vi "ME_acquire_3.vi"() -> ()   [LabVIEW 2015]
doc: "Use this template to build a producer/consumer design pattern. Use this template when you need to execute a process, such as data analysis, when a data source, such as a triggered acquisition, produces data at an uneven rate and you need to execute the process when the data becomes available."
uses:
  oxford_driver/Oxford Drivers/BUSGEN.LLB/OxfordAddress.ctl
  <vilib>/gmath/NI_Gmath.lvlib
  <vilib>/Utility/file.llb/Write Delimited Spreadsheet (DBL).vi
  <vilib>/express/express arith-compare/Formula/XNode/ExpressFormulaBlockNode.xnode
panel:
  out "I_dn_average":dbl[](array[numeric]) format="%_6g"
  out "I_dn_actual":dbl[](array[numeric]) format="%_6g"
  out "B array":dbl[](array[numeric])
  in  "dB (T)":dbl=0.0001
  in  "Counter":dbl
  out "I(B) 3":cluster{dbl[], dbl[]}(graph)
  out "I(B) 2":cluster{dbl[], dbl[]}(graph)
  out "I(B)":cluster{dbl[], dbl[]}(graph)
  in  "Max Field (T)":dbl
  in  "Min Field (T)":dbl
  in  "Ramp up/down":bool
  out "I_T":cluster{dbl[], dbl[]}(graph)
  in  "Field To Zero":bool
  in  "Set Field (T)":dbl=0.3
  in  "Go to Set":bool
  out "L magnet (H)":dbl
  out "R magnet (mOhm)":dbl
  out "Actual Current (R0)":dbl
  out "Actual Field (T)":dbl
  out "Set":bool
  in  "Target Sweep Rate (T/min)":dbl=2.0 format="%.6f"
  out "Temperature array":dbl[](array[numeric])
  in  "New Measurement File":bool
  out "Measurement File":path
  out "refnum out":refnum<file>
  in  "Sampling rate (Hz)":dbl=20.0
  in  "Measuring":bool
  out "Actual Temperature (K)":dbl
  in  "Temp Refresh (s)":dbl=1.0
  in  "Lake Shore":refnum<visa-resource-name>="GPIB0::11::INSTR"
  out "Time Lag":dbl=0.0500025749206543
  out "Magnetic Field":cluster{dbl[], dbl[]}(graph)
  out "IV converter":cluster{dbl[], dbl[]}(graph)
  in  "Measure (Start/Pause)":bool
  in  "Magnetic Field":refnum<visa-resource-name>="GPIB0::21::INSTR"
  in  "IV converter":refnum<visa-resource-name>="GPIB0::20::INSTR"
  in  "stop":bool
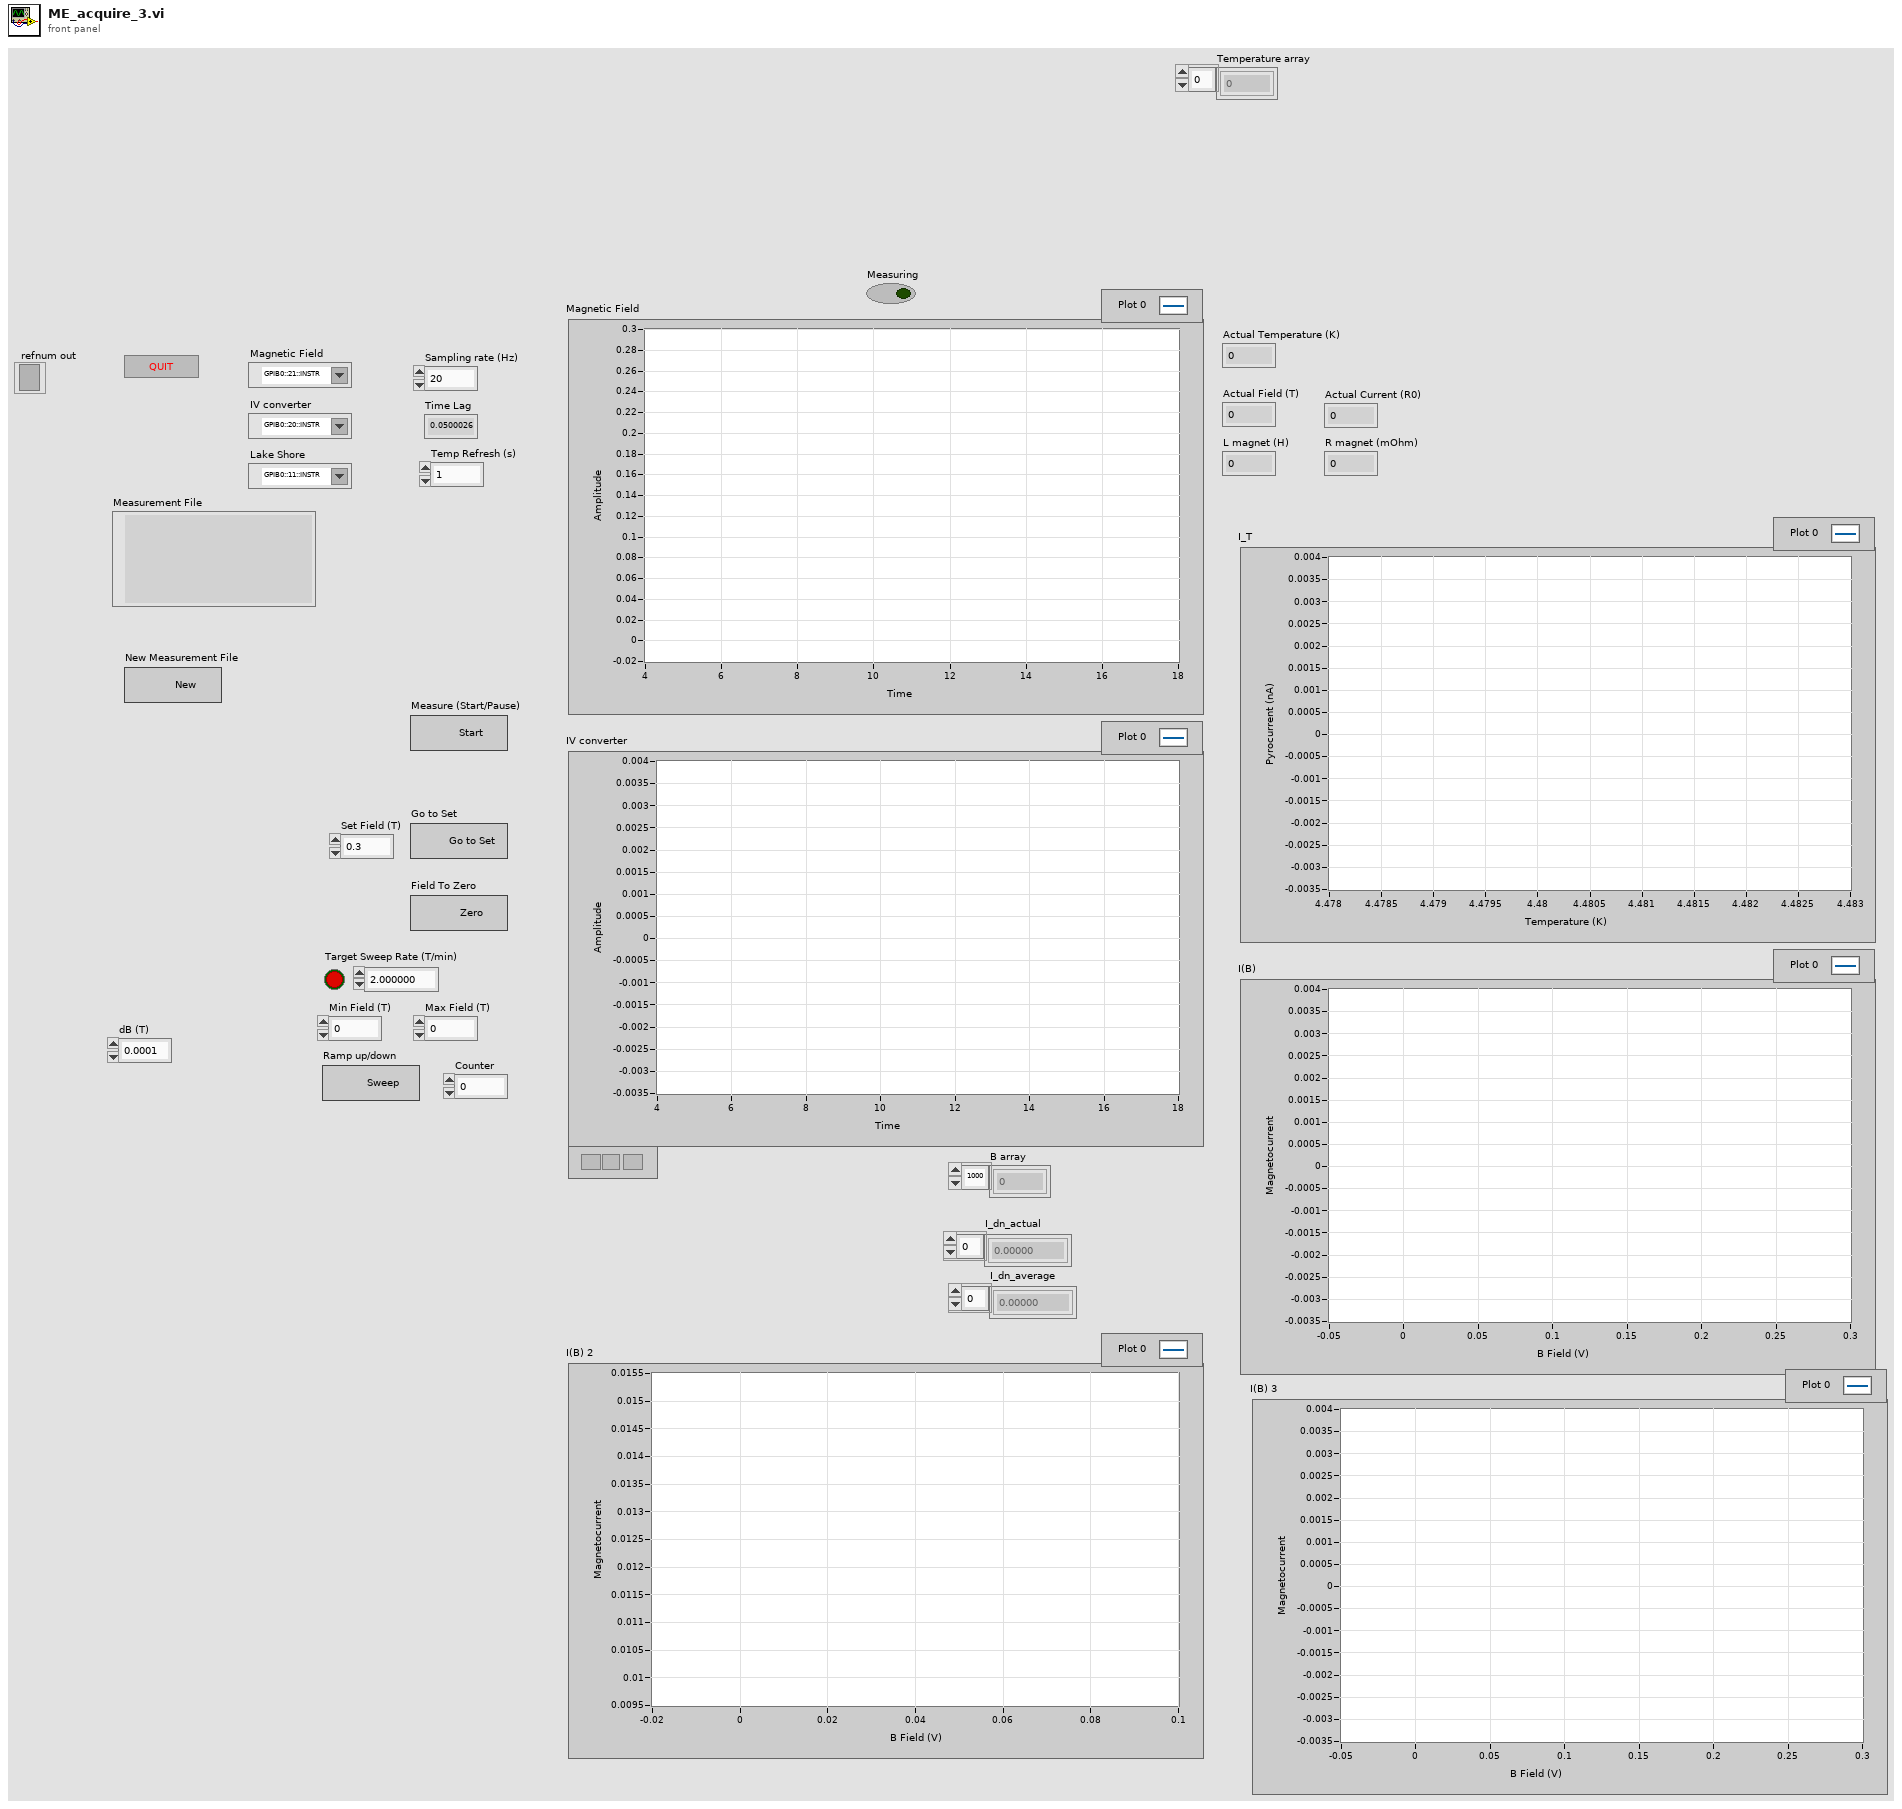
[diagram p1: front panel]
types:
  T1 = enum16{"open", "replace", "create", "open or create", "replace or create", "replace or create with confirmation"}
  T2 = typedef "OxfordAddress.ctl" = cluster{"Com Port":i32, "ISOBUS Address":i32, "GPIB Address":i16, "Communication":enum16{"RS232", "ISOBUS", "GPIB", "Gateway"}}
  T3 = cluster{"seconds since 1Jan1904":timestamp, "read buffer":string, "read buffer":string}
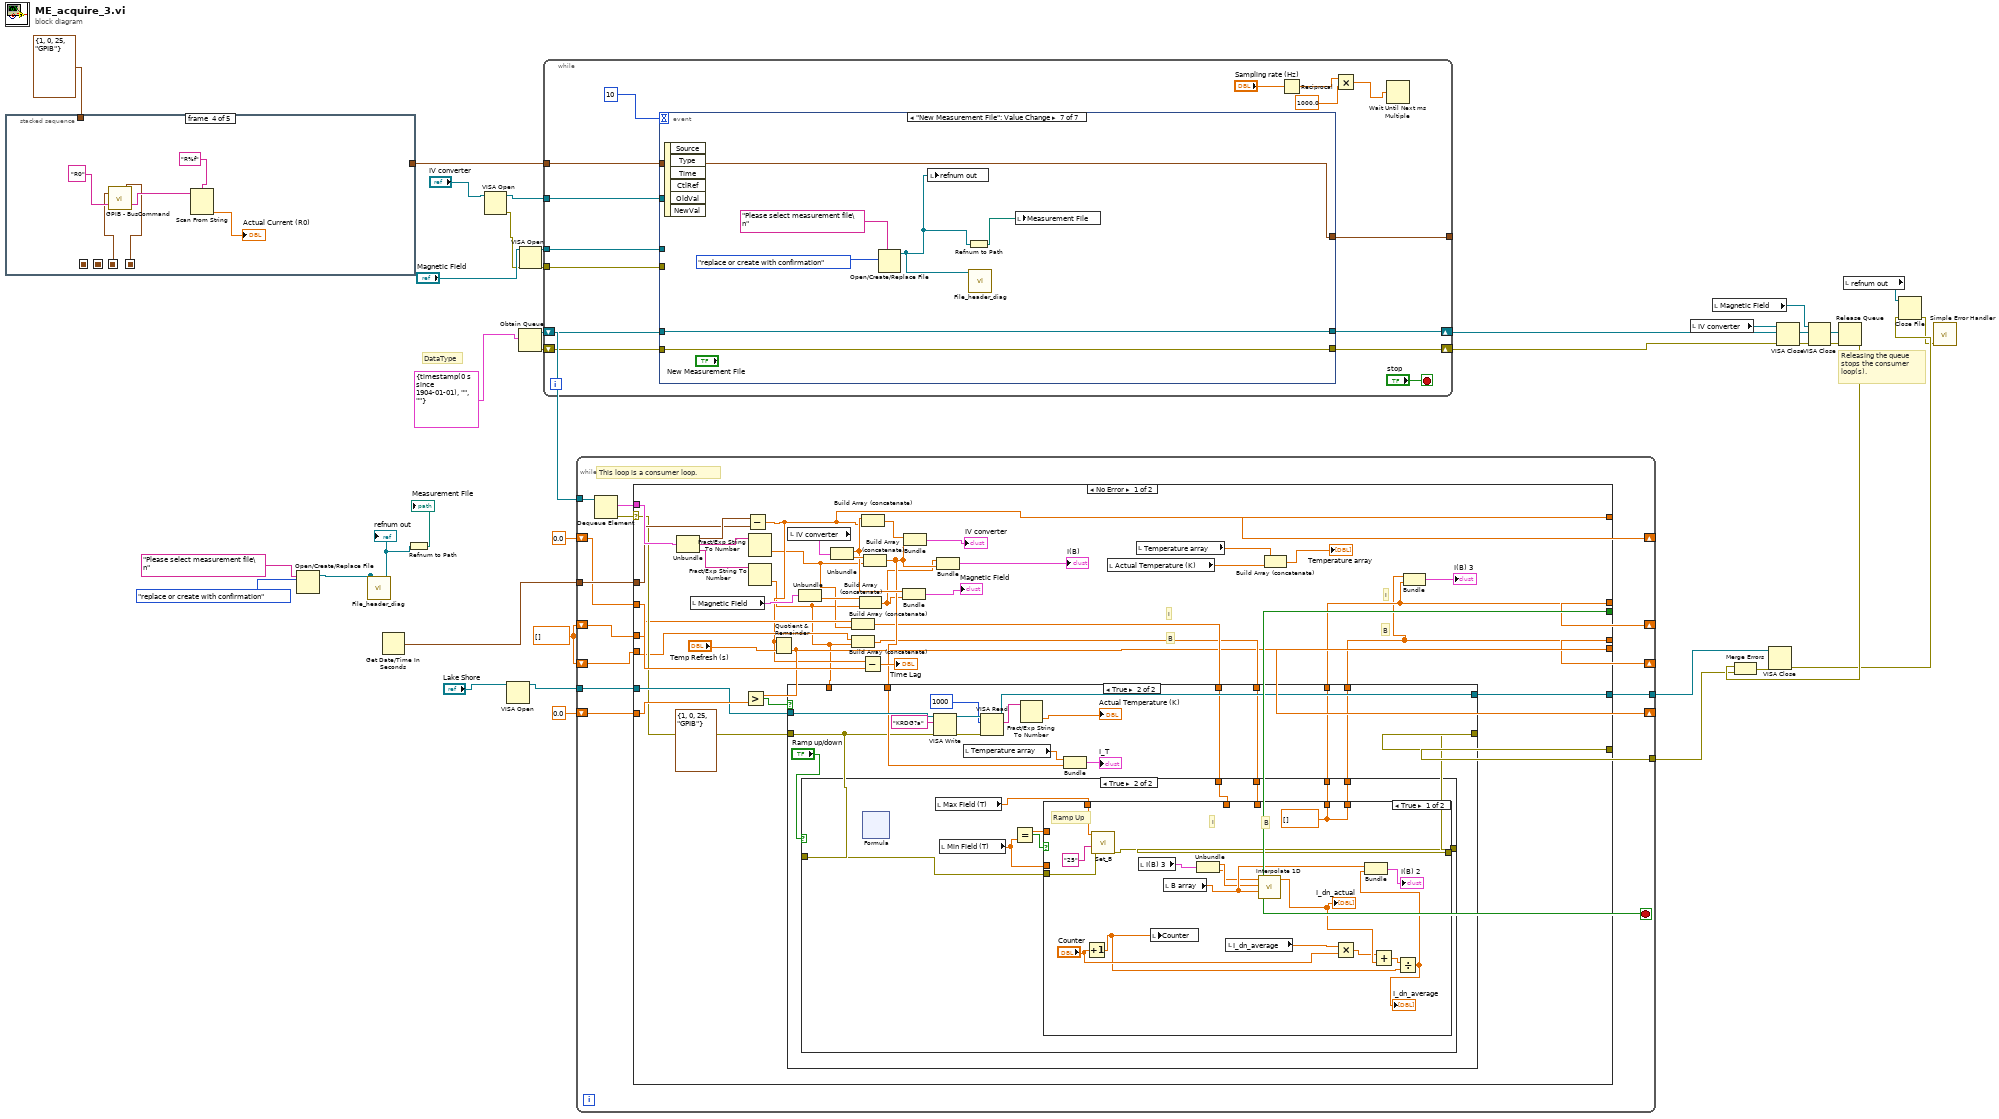
[diagram p0: block diagram]
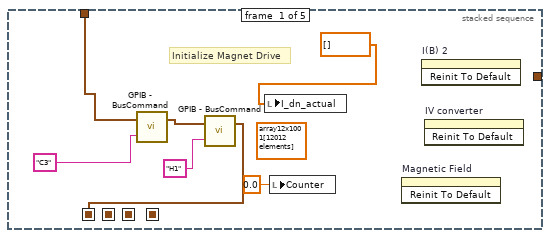
[diagram p2: hidden frame]
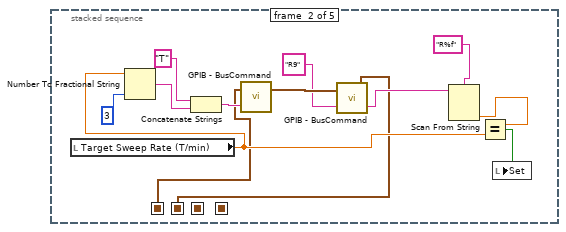
[diagram p3: hidden frame]
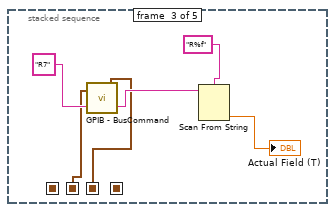
[diagram p4: hidden frame]
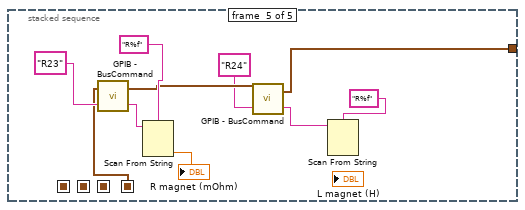
[diagram p5: hidden frame]
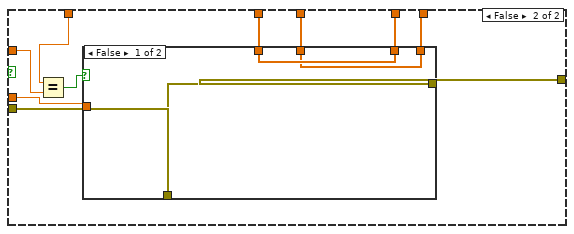
[diagram p8: hidden frame]
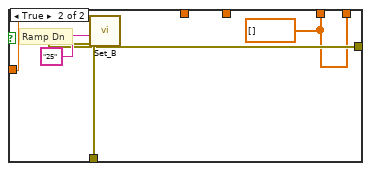
[diagram p9: hidden frame]
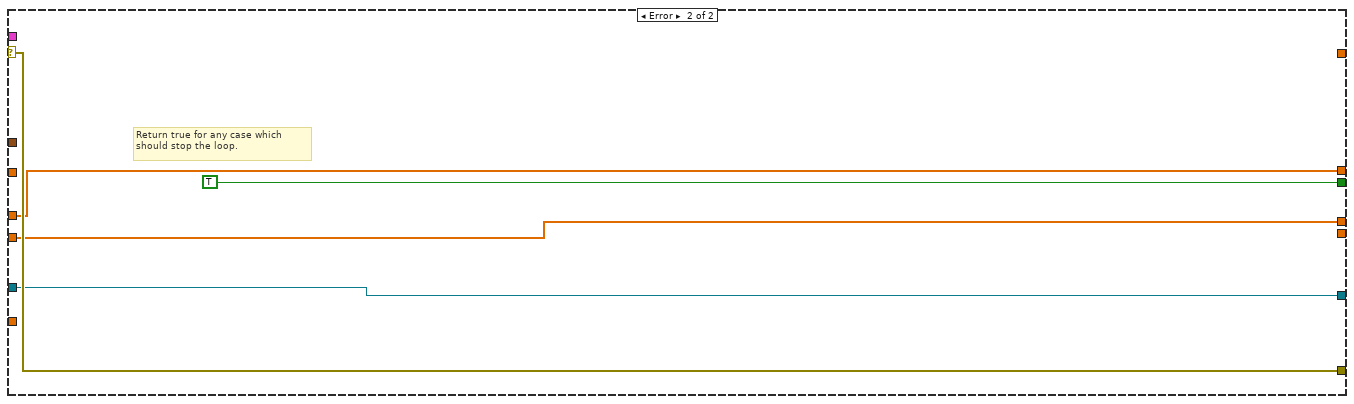
[diagram p10: hidden frame]
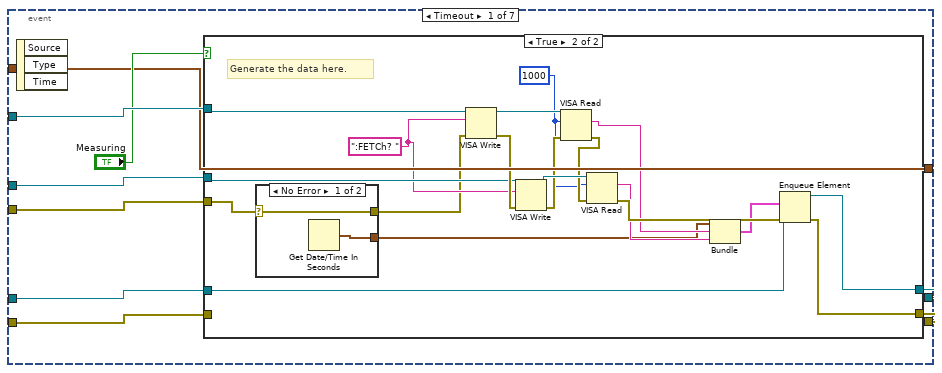
[diagram p11: hidden frame]
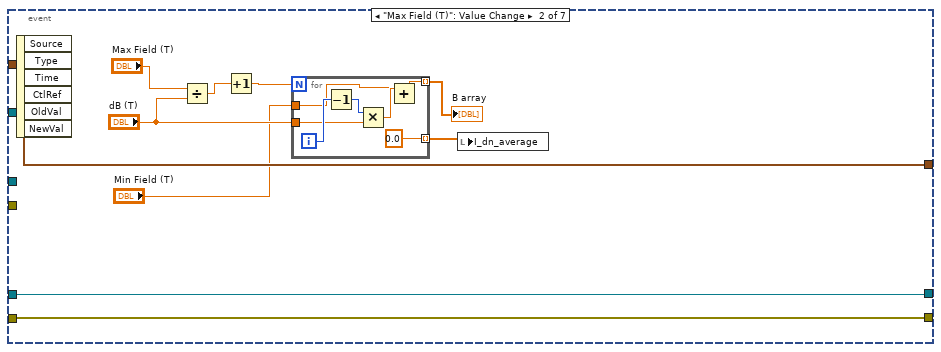
[diagram p14: hidden frame]
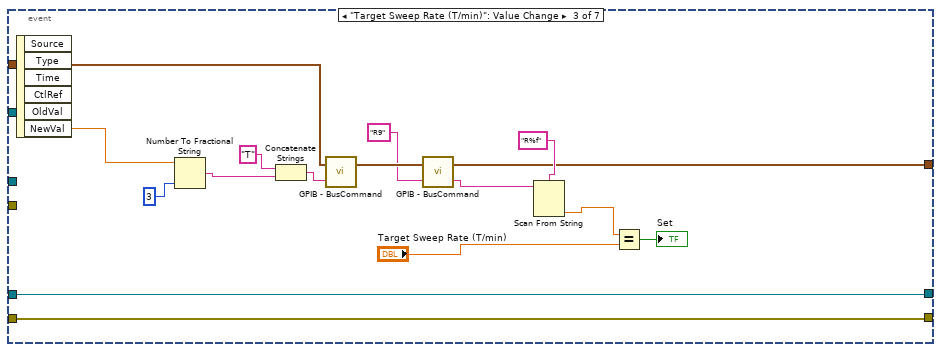
[diagram p15: hidden frame]
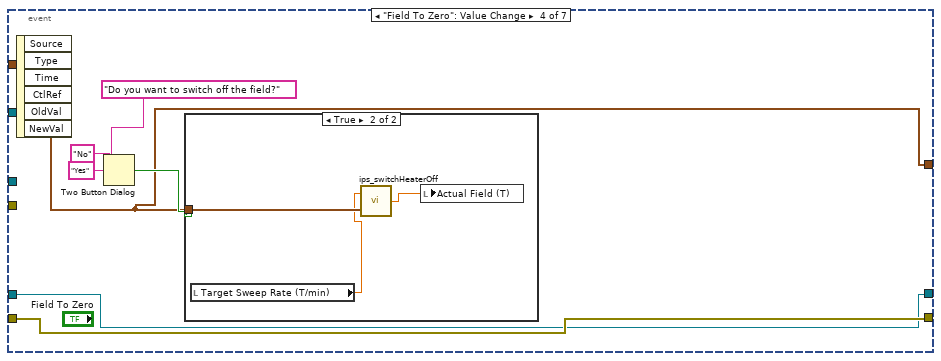
[diagram p16: hidden frame]
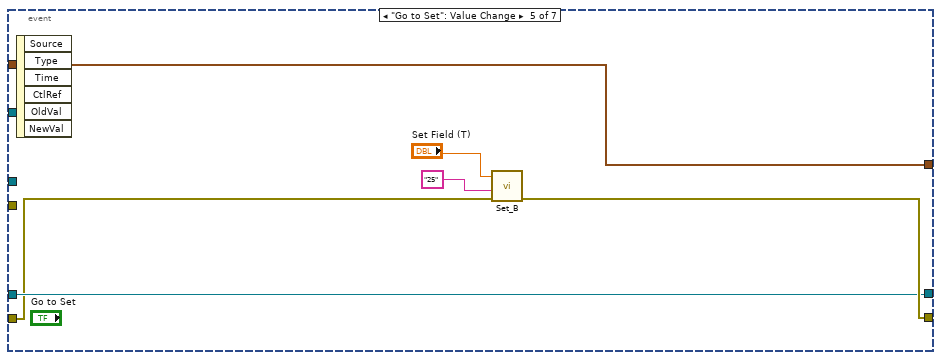
[diagram p18: hidden frame]
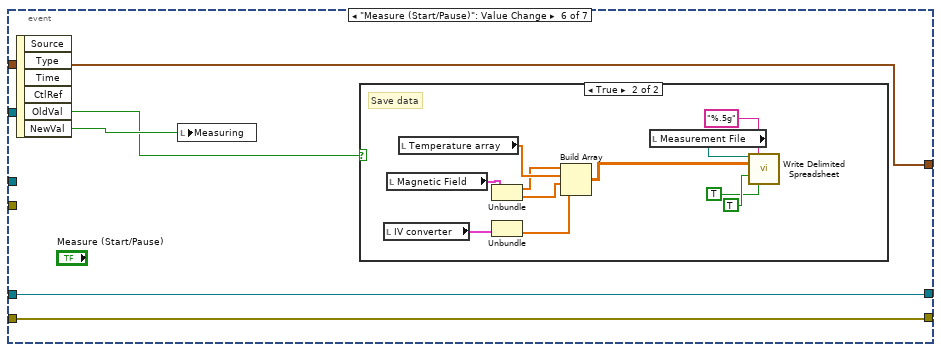
[diagram p19: hidden frame]
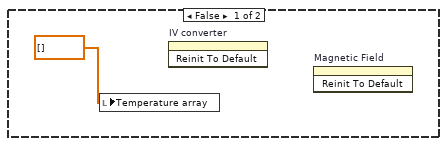
[diagram p20: hidden frame]
diagram:
  w5 = dbl[] []
  # "DataType"
  # "Releasing the queue stops the consumer loop(s)."
  n1 = stacked-sequence {
    seq-local: [w37 _ _ _ _] -> [_ w43 _ _ _]
    seq-local: [_ w42 _ _ _] -> [_ _ w56 _ _]
    seq-local: [_ _ w55 _ _] -> [_ _ _ w62 _]
    seq-local: [_ _ _ w61 _] -> [_ _ _ _ w72]
    tunnel: T2 {"Com Port"=1, "ISOBUS Address"=0, "GPIB Address"=25, "Communication"=enum."GPIB"} ("Address") -> [w40 _ _ _ _]
    tunnel: [_ _ _ _ w70] -> w6
    frame #0 {
      (unwired) dbl[][] array12x1001[12012 elements] ("I_dn_all")
      # "Initialize Magnet Drive"
      n2 = call "GPIB - BusCommand.vi"("Command"="C3", "Address"=w40) -> ("Address(thru)"=w38:T2)  [unwired: 1 out]
      n3 = call "GPIB - BusCommand.vi"("Command"="H1", "Address"=w38) -> ("Address(thru)"=w37:T2)  [unwired: 1 out]
      n4 = local write "I_dn_actual"(dbl[] [] ("Result")) -> ()
      n5 = local write "Counter"(0.0 ("Counter")) -> ()
      n6 = invoke on="Magnetic Field" class="XYGraph (strict)" method="Reinit To Default"() -> ()  [unwired: 3 in, 3 out]
      n7 = invoke on="I(B) 2" class="XYGraph (strict)" method="Reinit To Default"() -> ()  [unwired: 3 in, 3 out]
      n8 = invoke on="IV converter" class="XYGraph (strict)" method="Reinit To Default"() -> ()  [unwired: 3 in, 3 out]
    }
    frame #1 {
      n9 = local read "Target Sweep Rate (T/min)"() -> (w45:dbl)
      n10 = Number To Fractional String(number=w45, precision (6)=i16 3) -> (F-format string=w52:string)  [unwired: 2 in]
      n11 = Concatenate Strings("T" ("format string"), w52) -> (w51:string)
      n12 = call "GPIB - BusCommand.vi"("Command"=w51, "Address"=w43) -> ("Address(thru)"=w50:T2)  [unwired: 1 out]
      n13 = call "GPIB - BusCommand.vi"("Command"="R9" ("format string"), "Address"=w50) -> ("Reply"=w48:string, "Address(thru)"=w42:T2)
      n14 = Scan From String(format string="R%f" ("remaining string"), input string=w48) -> (output 1=w46:dbl)  [unwired: 3 in, 3 out]
      n15 = Equal?(x=w46, y=w45) -> (x = y?=w44:bool)
      n16 = local write "Set"(w44) -> ()
    }
    frame #2 {
      n17 = call "GPIB - BusCommand.vi"("Command"="R7" ("format string"), "Address"=w56) -> ("Reply"=w60:string, "Address(thru)"=w55:T2)
      n18 = Scan From String(format string="R%f" ("remaining string"), input string=w60) -> (output 1=→"Actual Field (T)":dbl)  [unwired: 3 in, 3 out]
    }
    frame #3 {
      n19 = call "GPIB - BusCommand.vi"("Command"="R0" ("format string"), "Address"=w62) -> ("Reply"=w66:string, "Address(thru)"=w61:T2)
      n20 = Scan From String(format string="R%f" ("remaining string"), input string=w66) -> (output 1=→"Actual Current (R0)":dbl)  [unwired: 3 in, 3 out]
    }
    frame #4 {
      n21 = call "GPIB - BusCommand.vi"("Command"="R23" ("format string"), "Address"=w72) -> ("Reply"=w76:string, "Address(thru)"=w71:T2)
      n22 = Scan From String(format string="R%f" ("remaining string"), input string=w76) -> (output 1=→"R magnet (mOhm)":dbl)  [unwired: 3 in, 3 out]
      n23 = call "GPIB - BusCommand.vi"("Command"="R24" ("format string"), "Address"=w71) -> ("Reply"=w68:string, "Address(thru)"=w70:T2)
      n24 = Scan From String(format string="R%f" ("remaining string"), input string=w68) -> ()  [unwired: 4 in, 3 out]
    }
  }
  n25 = Open/Create/Replace File(prompt="Please select measurement file\n", operation (0:open)=T1."replace or create with confirmation") -> (refnum out=w1:refnum<file>)  [unwired: 4 in, 2 out]
  "refnum out" <- w1
  n26 = call "File_header_diag.vi"("Byte Stream File in"=w1) -> ()  [unwired: 11 in]
  n27 = Get Date/Time In Seconds() -> (seconds since 1Jan1904=w19:timestamp)
  n28 = Refnum to Path(1:w1) -> (0:→"Measurement File":path)
  n29 = VISA Open(VISA resource name="IV converter") -> (VISA resource name=w28:refnum<visa-resource-name>, error out=w30:errorcluster)  [unwired: 4 in]
  n30 = VISA Open(VISA resource name="Lake Shore") -> (VISA resource name=w17:refnum<visa-resource-name>)  [unwired: 4 in, 1 out]
  n31 = Obtain Queue(element data type=T3 {"seconds since 1Jan1904"=timestamp(0 s since 1904-01-01), "read buffer"="", "read buffer"=""} ("output cluster")) -> (queue out=w34:refnum<queue>, error out=w33:errorcluster)  [unwired: 4 in, 1 out]
  n32 = VISA Open(error in (no error)=w30, VISA resource name="Magnetic Field") -> (VISA resource name=w27:refnum<visa-resource-name>, error out=w26:errorcluster)  [unwired: 3 in]
  n33 = while {
    shift-right: [w87] -> w24
    shift-left: w33 -> [w88]
    shift-right: [w89] -> w32
    shift-left: w34 -> [w90]
    tunnel: w28 -> [w86]
    tunnel: w27 -> [w85]
    tunnel: w26 -> [w84]
    tunnel: [w78] -> _
    tunnel: w6 -> [w77]
    stop <- "stop" stop-if-true
    n34 = event shown="[6] \"New Measurement File\": Value Change" {
      selector: _ -> [_ _ _ _ _ _ _]
      dyn-events: _ -> [_ _ _ _ _ _ _]
      timeout: 10 -> [_ _ _ _ _ _ _]
      tunnel: w90 -> [w100 w134 w143 w159 w170 w178 w192]
      tunnel: [w99 w134 w143 w159 w170 w178 w192] -> w89
      tunnel: w88 -> [w98 w133 w142 w160 w169 w177 w193]
      tunnel: [w97 w133 w142 w160 w171 w177 w193] -> w87
      tunnel: w86 -> [w96 _ _ _ _ _ _]
      tunnel: w85 -> [w95 _ _ _ _ _ _]
      tunnel: w84 -> [w94 _ _ _ _ _ _]
      tunnel: [w92 w132 w148 w158 w172 w174 w191] -> w78
      tunnel: w77 -> [w92 w132 w144 w158 w172 w174 w191]
      event Timeout {
        n35 = event-data() -> ()  [unwired: 1 in, 3 out]
        n36 = case shown="True" "Measuring" {
          tunnel: w100 -> [w102 w121]
          tunnel: [w102 w120] -> w99
          tunnel: w98 -> [w101 _]
          tunnel: [w101 w119] -> w97
          tunnel: w96 -> [_ w112]
          tunnel: w95 -> [_ w111]
          tunnel: w94 -> [_ w106]
          frame False {
          }
          frame True {
            w109 = ":FETCh? " ("data")
            w113 = u32 1000 ("byte count")
            # "Generate the data here."
            n37 = case shown="No Error" w106 {
              selector: w106 -> [w123 w124]
              tunnel: [w123 w124] -> w105
              tunnel: [w122 _] -> w104
              frame No Error {
                n38 = Get Date/Time In Seconds() -> (seconds since 1Jan1904=w122:timestamp)
              }
              frame Error {
              }
            }
            n39 = VISA Write(VISA resource name=w112, write buffer=w109, error in (no error)=w105) -> (VISA resource name out=w118:refnum<visa-resource-name>, error out=w116:errorcluster)  [unwired: 1 out]
            n40 = VISA Write(VISA resource name=w111, write buffer=w109, error in (no error)=w116) -> (VISA resource name out=w117:refnum<visa-resource-name>, error out=w115:errorcluster)  [unwired: 1 out]
            n41 = VISA Read(VISA resource name=w118, byte count=w113, error in (no error)=w115) -> (read buffer=w107:string, error out=w114:errorcluster)  [unwired: 2 out]
            n42 = VISA Read(VISA resource name=w117, byte count=w113, error in (no error)=w114) -> (read buffer=w108:string, error out=w110:errorcluster)  [unwired: 2 out]
            n43 = Bundle("seconds since 1Jan1904"=w104, "read buffer"=w107, "read buffer"=w108) -> (w103:T3)  [unwired: 1 in]
            n44 = Enqueue Element(queue=w121, element=w103, error in (no error)=w110) -> (queue out=w120:refnum<queue>, error out=w119:errorcluster)  [unwired: 1 in, 1 out]
          }
        }
      }
      event "Max Field (T)": Value Change {
        n45 = event-data() -> ()  [unwired: 1 in, 6 out]
        n46 = Divide(x="Max Field (T)", y="dB (T)") -> (x/y=w129:dbl)
        n47 = Increment(x=w129) -> (x+1=w128:dbl)
        n48 = for {
          N: w128 -> [_]
          tunnel: "dB (T)" -> [w139]
          tunnel: [w136] -> w127 mode=indexing
          tunnel: "Min Field (T)" -> [w137]
          tunnel: [0.0] -> w125 mode=indexing
          i -> [w141]
          n49 = Decrement(x=w141) -> (x-1=w140:i32)
          n50 = Multiply(x=w140, y=w139) -> (x*y=w138:dbl)
          n51 = Add(x=w138, y=w137) -> (x+y=w136:dbl)
        }
        "B array" <- w127
        n52 = local write "I_dn_average"(w125) -> ()
      }
      event "Target Sweep Rate (T/min)": Value Change {
        n53 = event-data() -> ("NewVal"=w156:dbl)  [unwired: 1 in, 5 out]
        n54 = Number To Fractional String(number=w156, precision (6)=i16 3) -> (F-format string=w154:string)  [unwired: 2 in]
        n55 = Concatenate Strings("T" ("format string"), w154) -> (w153:string)
        n56 = call "GPIB - BusCommand.vi"("Command"=w153, "Address"=w144) -> ("Address(thru)"=w152:T2)  [unwired: 1 out]
        n57 = call "GPIB - BusCommand.vi"("Command"="R9" ("format string"), "Address"=w152) -> ("Reply"=w150:string, "Address(thru)"=w148:T2)
        n58 = Scan From String(format string="R%f" ("remaining string"), input string=w150) -> (output 1=w147:dbl)  [unwired: 3 in, 3 out]
        n59 = Equal?(x=w147, y="Target Sweep Rate (T/min)") -> (x = y?=→"Set":bool)
      }
      event "Field To Zero": Value Change {
        n60 = event-data() -> ()  [unwired: 1 in, 6 out]
        n61 = Two Button Dialog(message="Do you want to switch off the field?", 1:"No" ("F button name (\"Cancel\")"), 2:"Yes" ("T button name (\"OK\")")) -> (T button?=w164:bool)
        n62 = case shown="True" w164 {
          tunnel: w158 -> [_ w167]
          frame False {
          }
          frame True {
            n63 = local read "Target Sweep Rate (T/min)"() -> (w166:dbl)
            n64 = call "ips_switchHeaterOff.vi"("Instrument address"=w167, "Rate"=w166) -> ("B"=w165:dbl)
            n65 = local write "Actual Field (T)"(w165) -> ()
          }
        }
      }
      event "Go to Set": Value Change {
        n66 = event-data() -> ()  [unwired: 1 in, 6 out]
        n67 = call "Set_B.vi"("error in (no error)"=w169, "address string"="25", "Set Field (T)"="Set Field (T)") -> ("error out"=w171:errorcluster)  [unwired: 8 in]
      }
      event "Measure (Start/Pause)": Value Change {
        n68 = event-data() -> ("OldVal"=w175:bool, "NewVal"=w176:bool)  [unwired: 1 in, 4 out]
        n69 = local write "Measuring"(w176) -> ()
        n70 = case shown="True" w175 {
          frame False {
            n71 = local write "Temperature array"(dbl[] []) -> ()
            n72 = invoke on="IV converter" class="XYGraph (strict)" method="Reinit To Default"() -> ()  [unwired: 3 in, 3 out]
            n73 = invoke on="Magnetic Field" class="XYGraph (strict)" method="Reinit To Default"() -> ()  [unwired: 3 in, 3 out]
          }
          frame True {
            # "Save data"
            n74 = local read "IV converter"() -> (w185:cluster{dbl[], dbl[]})
            n75 = local read "Magnetic Field"() -> (w184:cluster{dbl[], dbl[]})
            n76 = local read "Temperature array"() -> (w190:dbl[])
            n77 = Unbundle(w184) -> (w183:dbl[], w182:dbl[])
            n78 = Unbundle(w185) -> (w181:dbl[])  [unwired: 1 out]
            n79 = Build Array(w183, w190, w182, w181) -> (w187:dbl[][])
            n80 = local read "Measurement File"() -> (w188:path)
            n81 = call-poly <vilib>:"Write Delimited Spreadsheet.vi"("file path (dialog if empty)"=w188, "format (%.3f)"="%.5g", "2D data"=w187, "append to file? (F)"=TRUE, "transpose? (F)"=TRUE) -> ()  [unwired: 9 in, 2 out]
          }
        }
      }
      event "New Measurement File": Value Change {
        n82 = event-data() -> ()  [unwired: 1 in, 6 out]
        n83 = Open/Create/Replace File(prompt="Please select measurement file\n", operation (0:open)=T1."replace or create with confirmation") -> (refnum out=w194:refnum<file>)  [unwired: 4 in, 2 out]
        n84 = local write "refnum out"(w194) -> ()
        n85 = Refnum to Path(1:w194) -> (0:w195:path)
        n86 = call "File_header_diag.vi"("Byte Stream File in"=w194) -> ()  [unwired: 11 in]
        n87 = local write "Measurement File"(w195) -> ()
      }
    }
    n88 = Reciprocal(x="Sampling rate (Hz)") -> (1/x=w82:dbl)
    n89 = Multiply(x=w82, y=1000.0) -> (x*y=w80:dbl)
    n90 = Wait Until Next ms Multiple(millisecond multiple=w80) -> ()  [unwired: 1 out]
  }
  n91 = while {
    tunnel: w34 -> [w213]
    tunnel: w19 -> [w209]
    shift-right: [w208] -> _
    shift-left: 0.0 -> [w207]
    tunnel: w17 -> [w206]
    shift-right: [w205] -> _
    shift-left: 0.0 -> [w204]
    tunnel: [w203] -> w11
    tunnel: [w202] -> w14
    shift-right: [w198] -> _
    shift-left: w5 -> [w201]
    shift-right: [w199] -> _
    shift-left: w5 -> [w200]
    stop <- w210 stop-if-true
    # "This loop is a consumer loop."
    n92 = Dequeue Element(queue=w213) -> (element=w211:T3, error out=w212:errorcluster)  [unwired: 2 in, 2 out]
    n93 = case shown="No Error" w212 {
      selector: w212 -> [w239 w334]
      tunnel: w211 -> [w252 _]
      tunnel: [_ TRUE] -> w210
      tunnel: w209 -> [w248 _]
      tunnel: [w217 _] -> w208
      tunnel: w207 -> [w245 _]
      tunnel: w206 -> [w240 w333]
      tunnel: [w220 _] -> w205
      tunnel: w204 -> [w242 _]
      tunnel: [w238 w334] -> w203
      tunnel: [w237 w333] -> w202
      tunnel: [w219 w331] -> w198
      tunnel: w201 -> [w224 w331]
      tunnel: w200 -> [w222 w332]
      tunnel: [w218 w332] -> w199
      frame No Error {
        (unwired) T2 {"Com Port"=1, "ISOBUS Address"=0, "GPIB Address"=25, "Communication"=enum."GPIB"} ("Address")
        # "B"
        # "I"
        # "I"
        # "B"
        n94 = Unbundle(w252) -> ("seconds since 1Jan1904"=w249:timestamp, "read buffer"=w251:string, "read buffer"=w250:string)
        n95 = local read "Magnetic Field"() -> (w233:cluster{dbl[], dbl[]})
        n96 = Subtract(x=w249, y=w248) -> (x-y=w217:dbl)
        n97 = Fract/Exp String To Number(string=w251) -> (number=w215:dbl)  [unwired: 3 in, 1 out]
        n98 = Fract/Exp String To Number(string=w250) -> (number=w214:dbl)  [unwired: 3 in, 1 out]
        n99 = Quotient & Remainder(x=w217, y="Temp Refresh (s)") -> (floor(x/y)=w220:dbl)  [unwired: 1 out]
        n100 = Greater?(x=w220, y=w242) -> (0:w241:bool)
        n101 = local read "IV converter"() -> (w231:cluster{dbl[], dbl[]})
        n102 = Unbundle(w233) -> (w232:dbl[])  [unwired: 1 out]
        n103 = Unbundle(w231) -> (w228:dbl[], w230:dbl[])
        n104 = Build Array (concatenate)(w224, w215) -> (w223:dbl[])
        n105 = Build Array (concatenate)(w222, w214) -> (w221:dbl[])
        n106 = Build Array (concatenate)(w232, w214) -> (w225:dbl[])
        n107 = Subtract(x=w217, y=w245) -> (x-y=→"Time Lag":dbl)
        n108 = Build Array (concatenate)(w228, w217) -> (w229:dbl[])
        n109 = Build Array (concatenate)(w230, w215) -> (w227:dbl[])
        n110 = case shown="True" w241 {
          tunnel: w240 -> [w255 w274]
          tunnel: w239 -> [w256 w263]
          tunnel: [w256 w262] -> w238
          tunnel: [w255 w268] -> w237
          tunnel: w227 -> [_ w265]
          tunnel: w223 -> [w253 w260]
          tunnel: w221 -> [w254 w259]
          tunnel: [w253 w258] -> w219
          tunnel: [w254 w257] -> w218
          tunnel: w214 -> [_ _]
          frame False {
          }
          frame True {
            n111 = case shown="True" "Ramp up/down" {
              tunnel: w263 -> [w277 w287]
              tunnel: [w277 w286] -> w262
              tunnel: w260 -> [w275 w281]
              tunnel: w259 -> [w276 w280]
              tunnel: [w275 w279] -> w258
              tunnel: [w276 w278] -> w257
              frame False {
              }
              frame True {
                n112 = xnode "Formula"() -> ()  [unwired: 2 in, 2 out]
                n113 = local read "Max Field (T)"() -> (w284:dbl)
                n114 = local read "Min Field (T)"() -> (w283:dbl)
                n115 = Equal?(x=w282, y=w283) -> (x = y?=w285:bool)
                n116 = case shown="True" w285 {
                  tunnel: w287 -> [w311 w322]
                  tunnel: [w309 w321] -> w286
                  tunnel: w284 -> [w310 w319]
                  tunnel: [_ w320] -> w282
                  tunnel: w283 -> [_ w318]
                  tunnel: w281 -> [_ w316]
                  tunnel: w280 -> [_ w314]
                  tunnel: [w308 w315] -> w279
                  tunnel: [w308 w313] -> w278
                  frame True {
                    w308 = dbl[] []
                    # "I"
                    # "B"
                    # "Ramp Up"
                    n117 = Increment(x="Counter") -> (x+1=w298:dbl)
                    n118 = call "Set_B.vi"("error in (no error)"=w311, "address string"="25", "Set Field (T)"=w310) -> ("error out"=w309:errorcluster)  [unwired: 8 in]
                    n119 = local read "I(B) 3"() -> (w306:cluster{dbl[], dbl[]})
                    n120 = local write "Counter"(w298) -> ()
                    n121 = local read "B array"() -> (w307:dbl[])
                    n122 = Unbundle(w306) -> (w305:dbl[], w304:dbl[])
                    n123 = local read "I_dn_average"() -> (w303:dbl[])
                    n124 = call <vilib>:"Interpolate 1D.vi"("xi"=w307, "X"=w305, "Y"=w304) -> ("yi"=w302:dbl[])  [unwired: 6 in, 2 out]
                    "I_dn_actual" <- w302
                    n125 = Multiply(x=w303, y="Counter") -> (x*y=w301:dbl[])
                    n126 = Add(x=w301, y=w302) -> (x+y=w299:dbl[])
                    n127 = Divide(x=w299, y=w298) -> (x/y=w296:dbl[])
                    "I_dn_average" <- w296
                    n128 = Bundle("B array"=w307, w296) -> (→"I(B) 2":cluster{"B array":dbl[], dbl[]})  [unwired: 1 in]
                  }
                  frame False {
                    n129 = Equal?(x=w319, y=w320) -> (x = y?=w317:bool)
                    n130 = case shown="False" w317 {
                      tunnel: w322 -> [w325 w329]
                      tunnel: [w325 w328] -> w321
                      tunnel: w318 -> [_ w327]
                      tunnel: w316 -> [w324 _]
                      tunnel: [w324 w326] -> w315
                      tunnel: w314 -> [w323 _]
                      tunnel: [w323 w326] -> w313
                      frame False {
                      }
                      frame True {
                        w326 = dbl[] []
                        # "Ramp Dn"
                        n131 = call "Set_B.vi"("error in (no error)"=w329, "address string"="25", "Set Field (T)"=w327) -> ("error out"=w328:errorcluster)  [unwired: 8 in]
                      }
                    }
                  }
                }
              }
            }
            n132 = VISA Write(VISA resource name=w274, write buffer="KRDG?a", error in (no error)=w263) -> (VISA resource name out=w272:refnum<visa-resource-name>, error out=w271:errorcluster)  [unwired: 1 out]
            n133 = local read "Temperature array"() -> (w266:dbl[])
            n134 = VISA Read(VISA resource name=w272, byte count=u32 1000, error in (no error)=w271) -> (VISA resource name out=w268:refnum<visa-resource-name>, read buffer=w269:string)  [unwired: 2 out]
            n135 = Fract/Exp String To Number(string=w269) -> (number=→"Actual Temperature (K)":dbl)  [unwired: 3 in, 1 out]
            n136 = Bundle("Temperature array"=w266, w265) -> (→"I_T":cluster{"Temperature array":dbl[], dbl[]})  [unwired: 1 in]
          }
        }
        n137 = Bundle(w228, w225) -> (→"Magnetic Field":cluster{dbl[], dbl[]})  [unwired: 1 in]
        n138 = Bundle(w229, w227) -> (→"IV converter":cluster{dbl[], dbl[]})  [unwired: 1 in]
        n139 = Bundle(w225, w227) -> (→"I(B)":cluster{dbl[], dbl[]})  [unwired: 1 in]
        n140 = local read "Actual Temperature (K)"() -> (w236:dbl)
        n141 = local read "Temperature array"() -> (w234:dbl[])
        n142 = Build Array (concatenate)(w234, w236) -> (→"Temperature array":dbl[])
        n143 = Bundle(w218, w219) -> (→"I(B) 3":cluster{dbl[], dbl[]})  [unwired: 1 in]
      }
      frame Error {
        # "Return true for any case which should stop the loop."
      }
    }
  }
  n144 = local read "IV converter"() -> (w22:refnum<visa-resource-name>)
  n145 = local read "Magnetic Field"() -> (w21:refnum<visa-resource-name>)
  n146 = VISA Close(VISA resource name=w22, error in (no error)=w24) -> (error out=w25:errorcluster)
  n147 = VISA Close(VISA resource name=w21, error in (no error)=w25) -> (error out=w23:errorcluster)
  n148 = Release Queue(queue=w32, error in (no error)=w23) -> (error out=w12:errorcluster)  [unwired: 1 in, 2 out]
  n149 = Merge Errors(w12, w11) -> (w13:errorcluster)
  n150 = VISA Close(VISA resource name=w14, error in (no error)=w13) -> (error out=w10:errorcluster)
  n151 = local read "refnum out"() -> (w8:refnum<file>)
  n152 = Close File(refnum=w8, error in=w10) -> (error out=w9:errorcluster)  [unwired: 1 out]
  n153 = call <vilib>:"Simple Error Handler.vi"("error in (no error)"=w9) -> ()  [unwired: 4 in, 5 out]
